vi "Cobro Prod.vi"(8 "error in (no error)":errorcluster, 11 "Productos in":refnum<class "Productos.lvclass">) -> (0 "error out":errorcluster, 3 "Productos out":refnum<class "Productos.lvclass">)   [LabVIEW 2020, in "Productos.lvlib" / "Productos.lvclass"]
uses:
  Productos.lvclass
  <vilib>/ActorFramework/Actor/Actor.lvclass
  UI Messages/Costo Update Msg/Costo Update Msg.lvclass
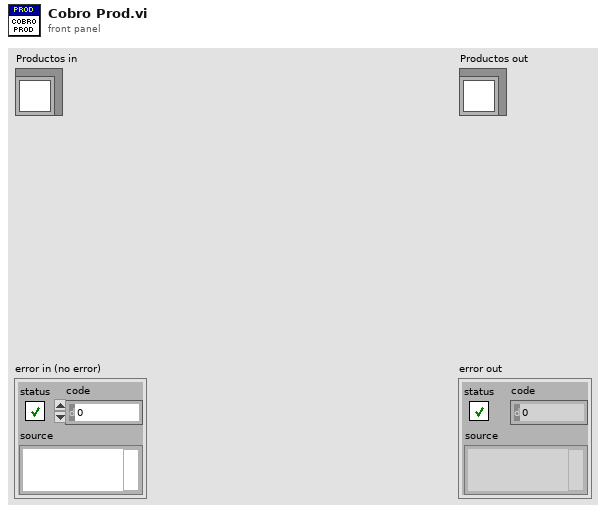
[diagram p1: front panel]
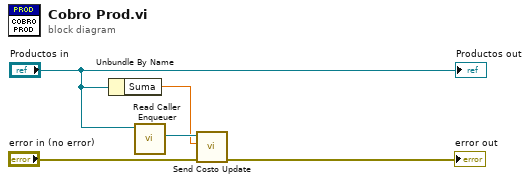
[diagram p0: block diagram]
diagram:
  n1 = Unbundle By Name("Productos in") -> ("Suma"=w3:dbl)
  n2 = call <vilib>:"Read Caller Enqueuer.vi"("Actor"="Productos in") -> ("Caller Enqueuer"=w4:refnum<class "Message Enqueuer.lvclass">)  [unwired: 10 in]
  n3 = call "Send Costo Update.vi"("error in (no error)"="error in (no error)", "Costo"=w3, "Message Enqueuer"=w4) -> ("error out"=→"error out":errorcluster)  [unwired: 7 in, 1 out]
  "Productos out" <- "Productos in"
